vi "TestWriteValue.vi"(8 "error in (no error)":errorcluster) -> (0 "error out":errorcluster)   [LabVIEW 2016]
uses:
  <vilib>/addons/_JKI Toolkits/Caraya/classes/Test/Test.lvclass
  <vilib>/addons/_JKI Toolkits/Caraya/classes/Assert/Assert.lvclass
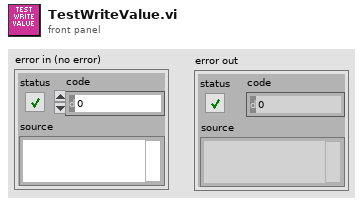
[diagram p1: front panel]
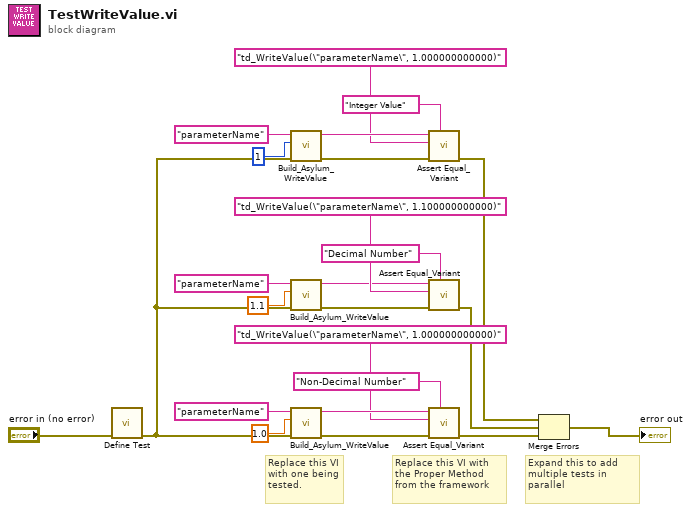
[diagram p0: block diagram]
diagram:
  # "Expand this to add multiple tests in parallel"
  # "Replace this VI with one being tested."
  # "Replace this VI with the Proper Method from the framework"
  n1 = call <vilib>:"Define Test.vi"("error in (no error)"="error in (no error)") -> ("error out"=w1:errorcluster)  [unwired: 10 in]
  n2 = call "Build_Asylum_WriteValue.vi"("error in (no error)"=w1, "value"=1, "parameterName"="parameterName") -> ("error out"=w7:errorcluster, "Command"=w6:string)  [unwired: 7 in]
  n3 = call "Build_Asylum_WriteValue.vi"("error in (no error)"=w1, "value"=1.1, "parameterName"="parameterName") -> ("error out"=w11:errorcluster, "Command"=w12:string)  [unwired: 7 in]
  n4 = call "Build_Asylum_WriteValue.vi"("error in (no error)"=w1, "value"=1.0, "parameterName"="parameterName") -> ("error out"=w20:errorcluster, "Command"=w19:string)  [unwired: 7 in]
  n5 = call <vilib>:"Assert Equal_Variant.vi"("Label"="Integer Value", "error in (no error)"=w7, "Y"="td_WriteValue(\"parameterName\", 1.000000000000)", "X"=w6) -> ("error out"=w2:errorcluster)  [unwired: 7 in]
  n6 = call <vilib>:"Assert Equal_Variant.vi"("Label"="Decimal Number", "error in (no error)"=w11, "Y"="td_WriteValue(\"parameterName\", 1.100000000000)", "X"=w12) -> ("error out"=w9:errorcluster)  [unwired: 7 in]
  n7 = call <vilib>:"Assert Equal_Variant.vi"("Label"="Non-Decimal Number", "error in (no error)"=w20, "Y"="td_WriteValue(\"parameterName\", 1.000000000000)", "X"=w19) -> ("error out"=w22:errorcluster)  [unwired: 7 in]
  n8 = Merge Errors(w2, w9, w22) -> (→"error out":errorcluster)
